vi "ApplyChannelSettings.vi"(8 "error in":errorcluster, 11 "Highland T564 DDG in":refnum<class "Highland T564 DDG.lvclass">) -> (0 "error out":errorcluster, 3 "Highland T564 DDG out":refnum<class "Highland T564 DDG.lvclass">)   [LabVIEW 2020, in "Highland T564 DDG.lvclass"]
uses:
  Highland T564 DDG.lvclass
  Channel.ctl
  Choice83.ctl
  Choice01.ctl
  Choice84.ctl
  T560Output.lvclass
  C:/GEECS/Developers Version/source/Device Drivers/Highland T564 DDG/SupportLibraries/DeviceSpecific/HighlandT560Lib/T560ChannelClass/T560Channel.lvclass
  Highland T564 DDG.lvclass/Highland T564 DDG.ctl
  T560Session.lvclass
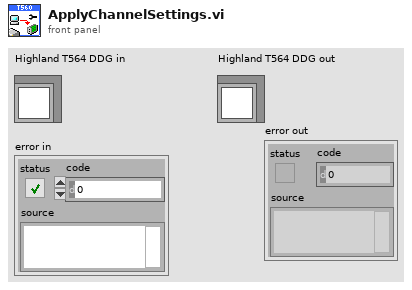
[diagram p1: front panel]
types:
  T1 = typedef "Channel.ctl" = cluster{"Polarity":T2, "ChannelOn":enum16{"off", "on"}, "Delay":T3, "Width":T3, "ChannelName":T4}
  T2 = typedef "Choice83.ctl" = enum16{"Direct", "Inverted"}
  T3 = typedef "Choice01.ctl" = cluster{"Value":dbl, "Min":dbl, "Max":dbl, "StepSize":dbl, "Tolerance":dbl, "ValueActual":dbl}
  T4 = typedef "Choice84.ctl" = enum16{"Null", "A", "B", "C", "D", "Trigger"}
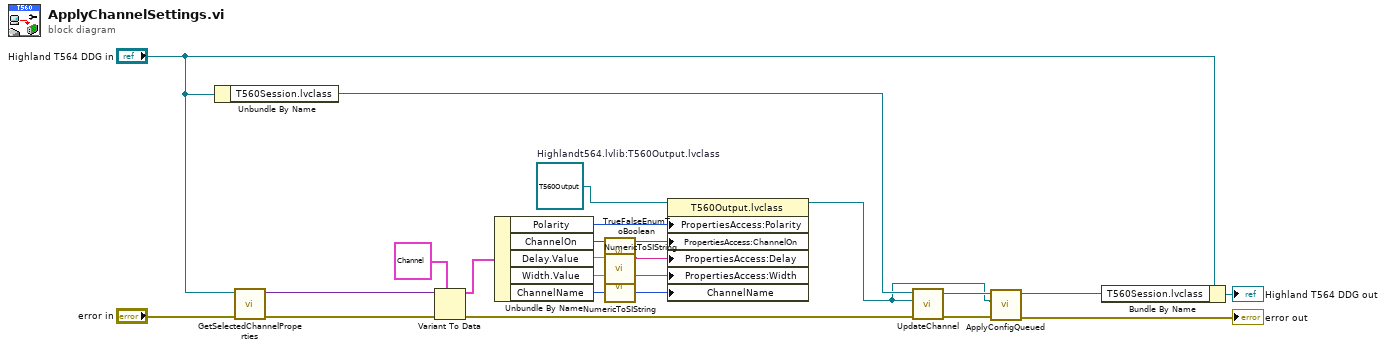
[diagram p0: block diagram]
diagram:
  w17 = refnum<class "T560Output.lvclass"> refnum  # Highlandt564.lvlib:T560Output.lvclass
  n1 = Unbundle By Name("Highland T564 DDG in") -> ("T560Session.lvclass"=w6:refnum<class "T560Session.lvclass">)
  n2 = call "GetSelectedChannelProperties.vi"("error in (no error)"="error in", "Highland T564 DDG in"="Highland T564 DDG in") -> ("error out"=w21:errorcluster, "ChannelProperties"=w19:variant)  [unwired: 8 in]
  n3 = Variant To Data(error in=w21, type=T1 {"Polarity"=enum."Direct", "ChannelOn"=enum."off", "Delay"={"Value"=0.0, "Min"=0.0, "Max"=0.0, "StepSize"=0.0, "Tolerance"=0.0, "ValueActual"=0.0}, "Width"={"Value"=0.0, "Min"=0.0, "Max"=0.0, "StepSize"=0.0, "Tolerance"=0.0, "ValueActual"=0.0}, "ChannelName"=enum."Null"} ("Settings.Channel1"), Variant=w19) -> (data=w18:T1, error out=w7:errorcluster)
  n4 = Unbundle By Name(w18) -> ("Polarity"=w16:T2, "ChannelOn"=w11:enum16{"off", "on"}, "Delay.Value"=w15:dbl, "Width.Value"=w13:dbl, "ChannelName"=w5:T4)
  n5 = call "TrueFalseEnumToBoolean.vi"("ChannelOn"=w11) -> ("selection"=w10:bool)  [unwired: 9 in, 1 out]
  n6 = call "NumericToSIString.vi"("Numeric"=w15) -> ("SI_String"=w14:string)  [unwired: 9 in, 1 out]
  n7 = call "NumericToSIString.vi"("Numeric"=w13) -> ("SI_String"=w12:string)  [unwired: 9 in, 1 out]
  n8 = property class="T560Output.lvclass"(reference=w17, "PropertiesAccess:Polarity"=w16, "PropertiesAccess:ChannelOn"=w10, "PropertiesAccess:Delay"=w14, "PropertiesAccess:Width"=w12, "ChannelName"=w5) -> (reference out=w1:refnum<class "T560Output.lvclass">)  [unwired: 1 in, 1 out]
  n9 = call-dynamic "UpdateChannel.vi"("error in"=w7, "UpdatedChannel.lvclass"=w1, "T560Session in"=w6) -> ("error out"=w9:errorcluster, "T560Session out"=w8:refnum<class "T560Session.lvclass">)  [unwired: 7 in]
  n10 = call-dynamic "ApplyConfigQueued.vi"("error in"=w9, "UpdatedChannel.lvclass"=w1, "T560Session in"=w8) -> ("error out"=→"error out":errorcluster, "T560Session out"=w4:refnum<class "T560Session.lvclass">)  [unwired: 7 in]
  n11 = Bundle By Name(cluster="Highland T564 DDG in", "T560Session.lvclass"=w4) -> (→"Highland T564 DDG out":refnum<class "Highland T564 DDG.lvclass">)
